vi "Create Child Actor.vi"(7 "App Inst":refnum<vi>, 8 "error in (no error)":errorcluster, 9 "Actor Name":string, 10 "Parent Class":refnum<vi>, 11 "Library in":refnum<vi>) -> (0 "error out":errorcluster, 3 "Library out":refnum<vi>)   [LabVIEW 2020, in "Add Actor.lvlib"]
uses:
  Add Actor.lvlib
  <vilib>/Utility/EditLVLibs/Edit LVLibs.lvlib
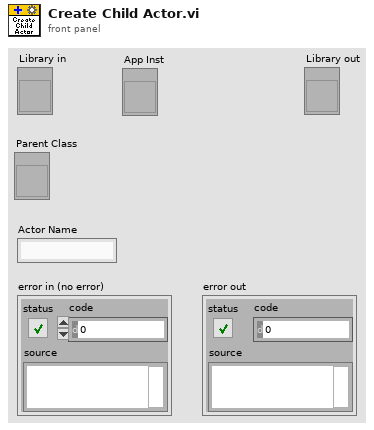
[diagram p1: front panel]
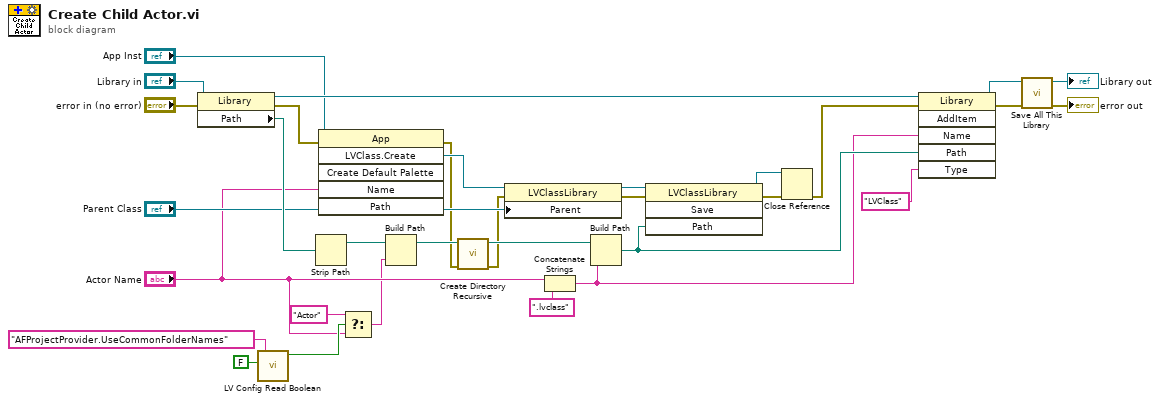
[diagram p0: block diagram]
diagram:
  n1 = property class="Library"(reference="Library in", error in="error in (no error)") -> (reference out=w30:refnum<vi>, error out=w23:errorcluster, "Path"=w27:path)
  n2 = call <resource>:"LV Config Read Boolean.vi"("default value"=FALSE, "key"="AFProjectProvider.UseCommonFolderNames") -> ("value"=w4:bool)  [unwired: 3 in, 2 out]
  n3 = Strip Path(path=w27) -> (stripped path=w17:path)  [unwired: 1 out]
  n4 = invoke class="App" method="LVClass.Create"(reference="App Inst", error in=w23, "Name"="Actor Name") -> (error out=w13:errorcluster, "LVClass.Create"=w22:refnum<vi>)  [unwired: 3 in, 4 out]
  n5 = Select(t="Actor", s=w4, f="Actor Name") -> (s? t:f=w1:string)
  n6 = Build Path(base path=w17, name or relative path=w1) -> (appended path=w15:path)
  n7 = call <vilib>:"Create Directory Recursive.vi"("error in (no error)"=w13, "directory"=w15) -> ("error out"=w12:errorcluster, "directory copy"=w14:path)  [unwired: 3 in, 1 out]
  n8 = property class="LVClassLibrary"(reference=w22, error in=w12, "Parent"="Parent Class") -> (reference out=w28:refnum<vi>, error out=w32:errorcluster)
  n9 = Concatenate Strings("Actor Name", ".lvclass" ("string")) -> (w16:string)
  n10 = Build Path(base path=w14, name or relative path=w16) -> (appended path=w25:path)
  n11 = invoke class="LVClassLibrary" method="Save"(reference=w28, error in=w32, "Path"=w25) -> (reference out=w21:refnum<vi>, error out=w20:errorcluster)  [unwired: 1 in, 2 out]
  n12 = Close Reference(reference=w21, error in (no error)=w20) -> (error out=w18:errorcluster)
  n13 = invoke class="Library" method="AddItem"(reference=w30, error in=w18, "Name"=w16, "Path"=w25, "Type"="LVClass") -> (reference out=w8:refnum<vi>, error out=w10:errorcluster)  [unwired: 1 in, 4 out]
  n14 = call <vilib>:"Save All This Library.vi"("error in (no error)"=w10, "Library in"=w8) -> ("error out"=→"error out":errorcluster, "Library out"=→"Library out":refnum<vi>)  [unwired: 8 in]
